vi "prepare dark model.vi"(8 "error in (no error)":errorcluster, 11 "Settings in":T1) -> (0 "error out":errorcluster)   [LabVIEW 2013, in "AvaSpec.lvlib" / "AvaSpec Logging.lvlib"]
uses:
  AvaSpec Logging.lvlib
  Settings/Settings.ctl
  Acquisition/Hardware Configuration.ctl
  Libraries/AS-5216-DLL/AVS settings.ctl
  Acquisition/Sphere Indicator.ctl
  Settings/Measurement Type.ctl
  Logging Configuration.ctl
  <vilib>/Analysis/baseanly.llb/Mean (DBL).vi
  <vilib>/Utility/file.llb/Write To Spreadsheet File (DBL).vi
  <vilib>/Analysis/NI_AALPro.lvlib
  <vilib>/Analysis/NI_AALBase.lvlib
  Settings/AvaSpec Settings.lvlib
  AvaSpec.lvlib
  Acquisition/AvaSpec Acquisition.lvlib
panel:
  out "Intercept Fit Verification":cluster{dbl[], "Best Power Fit":dbl[]}[](graph)
  out "Slope Fit Verification":cluster{dbl[], "Best Power Fit":dbl[]}[](graph)
  out "Offset Power model":dbl[](array[numeric])
  out "Slope Power model":dbl[](array[numeric])
  out "Average Residuals":dbl[](array[numeric])
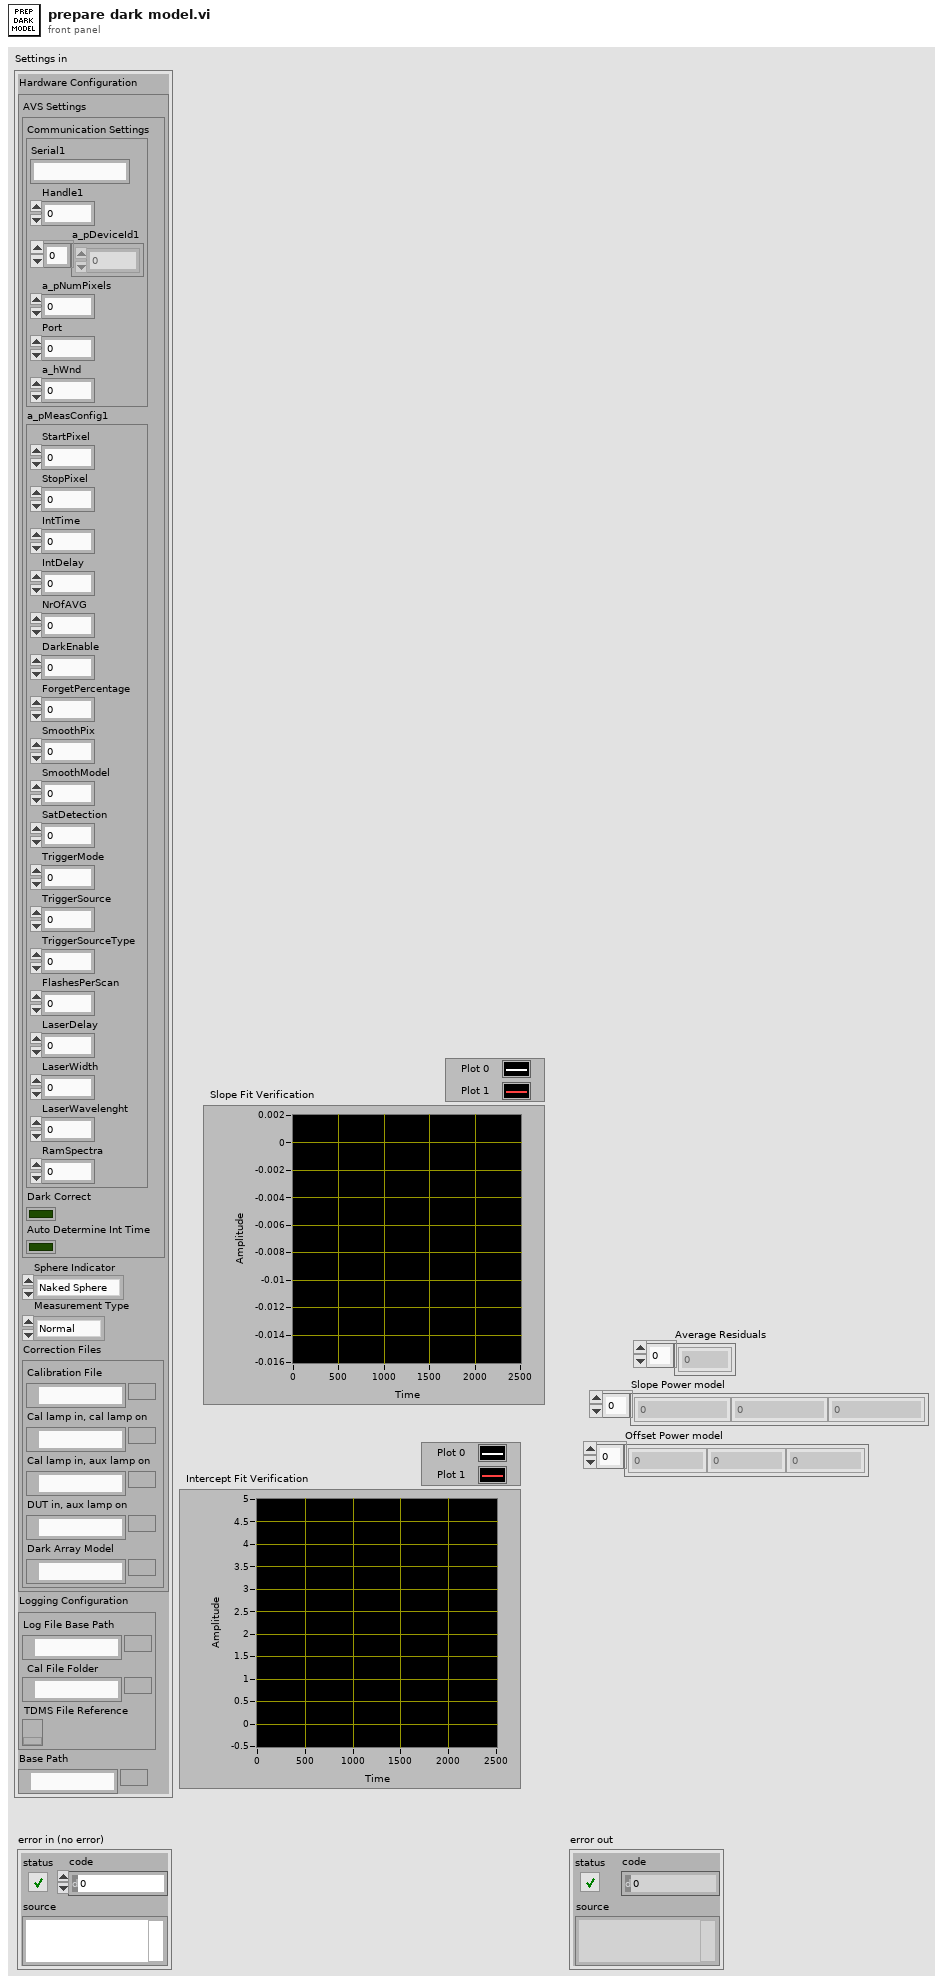
[diagram p1: front panel]
types:
  T1 = typedef "AvaSpec.lvlib/AvaSpec Settings.lvlib/Settings.ctl" = cluster{"Hardware Configuration":T2, "Logging Configuration":T6, "Base Path":path}
  T2 = typedef "AvaSpec.lvlib/AvaSpec Acquisition.lvlib/Hardware Configuration.ctl" = cluster{"AVS Settings":T3, "Sphere Indicator":T4, "Measurement Type":T5, "Correction Files":cluster{"Calibration File":path, "Cal lamp in, cal lamp on":path, "Cal lamp in, aux lamp on":path, "DUT in, aux lamp on":path, "Dark Array Model":path}}
  T3 = typedef "AvaSpec.lvlib/AVS settings.ctl" = cluster{"Communication Settings":cluster{"Serial1":string, "Handle1":i32, "a_pDeviceId1":u8[], "a_pNumPixels":u16, "Port":i32, "a_hWnd":i32}, "a_pMeasConfig1":cluster{"StartPixel":u16, "StopPixel":u16, "IntTime":sgl, "IntDelay":u32, "NrOfAVG":u32, "DarkEnable":u8, "ForgetPercentage":u8, "SmoothPix":u16, "SmoothModel":u8, "SatDetection":u8, "TriggerMode":u8, "TriggerSource":u8, "TriggerSourceType":u8, "FlashesPerScan":u16, "LaserDelay":u32, "LaserWidth":u32, "LaserWavelenght":sgl, "RamSpectra":u16}, "Dark Correct":bool, "Auto Determine Int Time":bool}
  T4 = typedef "AvaSpec.lvlib/Sphere Indicator.ctl" = enum16{"Naked Sphere", "Insulated Sphere"}
  T5 = typedef "AvaSpec.lvlib/AvaSpec Acquisition.lvlib/Measurement Type.ctl" = enum16{"Normal", "Calibration", "Dark"}
  T6 = typedef "AvaSpec.lvlib/AvaSpec Logging.lvlib/Logging Configuration.ctl" = cluster{"Log File Base Path":path, "Cal File Folder":path, "TDMS File Reference":refnum<k34>}
  T7 = cluster{"amp min":dbl, "amp max":dbl, "power min":dbl, "power max":dbl, "offset min":dbl, "offset max":dbl}
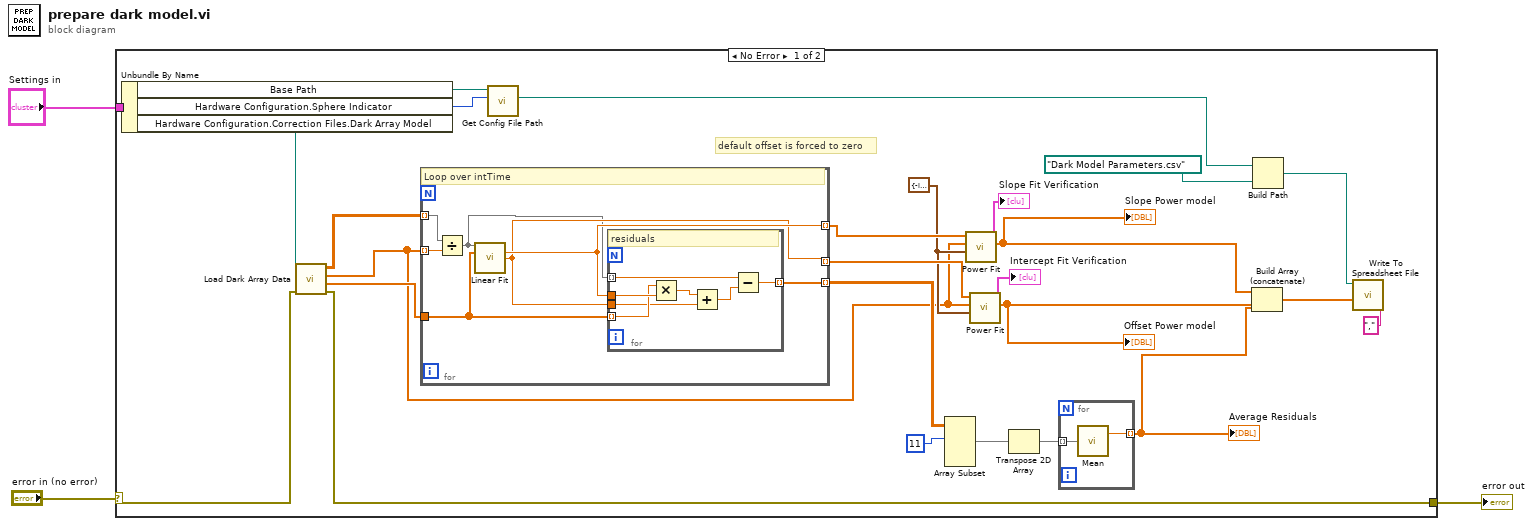
[diagram p0: block diagram]
diagram:
  n1 = case shown="No Error" "error in (no error)" {
    selector: "error in (no error)" -> [w5 w46]
    tunnel: [w4 w46] -> w2
    tunnel: "Settings in" -> [w12 _]
    frame No Error {
      w16 = T7 {"amp min"=-inf, "amp max"=inf, "power min"=-inf, "power max"=inf, "offset min"=-10.0, "offset max"=10.0} ("parameter bounds")
      # "default offset is forced to zero"
      n2 = Unbundle By Name(w12) -> ("Base Path"=w11:path, "Hardware Configuration.Sphere Indicator"=w10:T4, "Hardware Configuration.Correction Files.Dark Array Model"=w6:path)
      n3 = call "Load Dark Array Data.vi"("error in (no error)"=w5, "Dark Array Path"=w6) -> ("error out"=w4:errorcluster, "Freq"=w24:dbl[], "intTime"=w13:dbl[], "Scans"=w29:dbl[][])  [unwired: 6 in]
      n4 = for {
        tunnel: w29 -> [w35] mode=indexing
        tunnel: w13 -> [w33] mode=indexing
        tunnel: w24 -> [w38]
        tunnel: [w37] -> w23 mode=indexing
        tunnel: [w36] -> w17 mode=indexing
        tunnel: [w34] -> w28 mode=indexing
        # "Loop over intTime"
        n5 = Divide(x=w35, y=w33) -> (x/y=w32:dbl[])
        n6 = call <vilib>:"Linear Fit.vi"("Y"=w32, "X"=w38) -> ("slope"=w37:dbl, "intercept"=w36:dbl)  [unwired: 9 in, 3 out]
        n7 = for {
          tunnel: w38 -> [w44] mode=indexing
          tunnel: w37 -> [w45]
          tunnel: w36 -> [w42]
          tunnel: w32 -> [w40] mode=indexing
          tunnel: [w39] -> w34 mode=indexing
          # "residuals"
          n8 = Multiply(x=w44, y=w45) -> (x*y=w43:dbl)
          n9 = Add(x=w43, y=w42) -> (x+y=w41:dbl)
          n10 = Subtract(x=w40, y=w41) -> (x-y=w39:dbl)
        }
      }
      n11 = call "Get Config File Path.vi"("Sphere indicator"=w10, "Base Path"=w11) -> ("Cal File Folder"=w9:path)  [unwired: 7 in, 2 out]
      n12 = Array Subset(array=w28, index (row)=11 ("index")) -> (w20:dbl[][])  [unwired: 3 in]
      n13 = call "Power Fit.vi"("parameter bounds"=w16, "X"=w13, "Y"=w23) -> ("Power Model"=w27:dbl[], "Fit Verification"=→"Slope Fit Verification":cluster{dbl[], "Best Power Fit":dbl[]}[])  [unwired: 7 in]
      "Slope Power model" <- w27
      n14 = call "Power Fit.vi"("parameter bounds"=w16, "X"=w13, "Y"=w17) -> ("Power Model"=w14:dbl[], "Fit Verification"=→"Intercept Fit Verification":cluster{dbl[], "Best Power Fit":dbl[]}[])  [unwired: 7 in]
      "Offset Power model" <- w14
      n15 = Transpose 2D Array(2D array=w20) -> (transposed array=w19:dbl[][])
      n16 = for {
        tunnel: w19 -> [w31] mode=indexing
        tunnel: [w30] -> w18 mode=indexing
        n17 = call-poly <vilib>:"Mean.vi"("X"=w31) -> ("mean"=w30:dbl)  [unwired: 1 out]
      }
      "Average Residuals" <- w18
      n18 = Build Array (concatenate)(w27, w14, w18) -> (w26:dbl[])
      n19 = Build Path(base path=w9, name or relative path=path "Dark Model Parameters.csv" ("file path (dialog if empty)")) -> (appended path=w8:path)
      n20 = call-poly <vilib>:"Write To Spreadsheet File.vi"("delimiter (\\t)"="," ("delimiter (\\t)"), "1D data"=w26, "file path (dialog if empty)"=w8) -> ()  [unwired: 5 in, 1 out]
    }
    frame Error {
    }
  }
  "error out" <- w2
